vi "Update Hiden Scan Details.vi"(11 "Queue in":refnum<queue>) -> (3 "Queue Out":refnum<queue>)   [LabVIEW 2020]
uses:
  support/Message Queue/Message Cluster.ctl
  support/PCT FGV CMD.ctl
  <instrlib>/Hiden/Public/Scan/Scan Details.ctl
  <instrlib>/Hiden/Public/Scan/Scan Input Details.ctl
  <instrlib>/Hiden/Hiden MS.lvlib
  support/Message Queue/Message Queue.lvlib
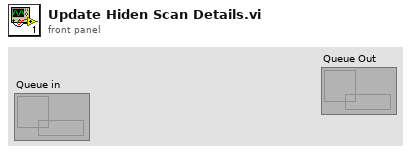
[diagram p1: front panel]
types:
  T1 = cluster{"Input device":string, "Autorange High":i16, "Autorange Low":i16, "Start range":i16, "Dwell (%)":u16, "Settle (%)":u16, "Boolean":bool, "Boolean":bool}
  T2 = typedef "PCT FGV CMD.ctl" = enum16{"INIT", "GET", "SET"}
  T3 = cluster{"Type CMD":string, "Mode CMD":string, "Main CMD":string}
  T4 = typedef "Hiden MS.lvlib/Scan Details.ctl" = cluster{"Device to scan":string, "Start value":dbl, "Stop value":dbl, "Increment":dbl}
  T5 = typedef "Hiden MS.lvlib/Scan Input Details.ctl" = cluster{"Input device":string, "Autorange High":i16, "Autorange Low":i16, "Start range":i16, "Dwell (%)":u16, "Settle (%)":u16, "Dwell is ms?":bool, "Settle is ms?":bool}
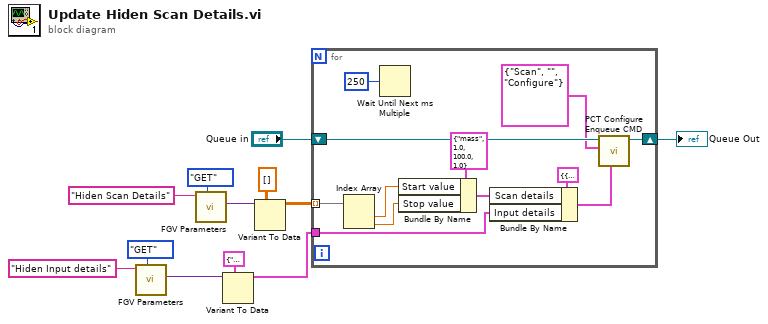
[diagram p0: block diagram]
diagram:
  n1 = call "FGV Parameters.vi"("CMD"=PCT_FGV_CMD."GET", "Key"="Hiden Input details") -> ("output"=w5:variant)  [unwired: 7 in, 2 out]
  n2 = call "FGV Parameters.vi"("CMD"=PCT_FGV_CMD."GET", "Key"="Hiden Scan Details") -> ("output"=w7:variant)  [unwired: 7 in, 2 out]
  n3 = Variant To Data(type=T1 {"Input device"="Faraday", "Autorange High"=-7, "Autorange Low"=-7, "Start range"=-7, "Dwell (%)"=100, "Settle (%)"=100, "Boolean"=FALSE, "Boolean"=FALSE} ("Hiden Input details"), Variant=w5) -> (data=w3:T1)  [unwired: 1 in, 1 out]
  n4 = Variant To Data(type=dbl[][] [] ("Hiden Scan Details"), Variant=w7) -> (data=w6:dbl[][])  [unwired: 1 in, 1 out]
  n5 = for {
    tunnel: w6 -> [w23] mode=indexing
    tunnel: w3 -> [w18]
    shift-right: [w13] -> w1
    shift-left: "Queue in" -> [w17]
    n6 = Index Array(array=w23) -> (element #1=w22:dbl, element #2=w21:dbl)  [unwired: 2 in]
    n7 = Wait Until Next ms Multiple(millisecond multiple=u32 250) -> ()  [unwired: 1 out]
    n8 = Bundle By Name(cluster=T4 {"Device to scan"="mass", "Start value"=1.0, "Stop value"=100.0, "Increment"=1.0} ("Scan details"), "Start value"=w22, "Stop value"=w21) -> (w19:T4)
    n9 = Bundle By Name(cluster=cluster{"Scan details":T4, "Input details":T5} {"Scan details"={"Device to scan"="mass", "Start value"=1.0, "Stop value"=100.0, "Increment"=1.0}, "Input details"={"Input device"="Faraday", "Autorange High"=-5, "Autorange Low"=-10, "Start range"=-7, "Dwell (%)"=100, "Settle (%)"=100, "Dwell is ms?"=FALSE, "Settle is ms?"=FALSE}} ("Scan Config"), "Scan details"=w19, "Input details"=w18) -> (w16:cluster{"Scan details":T4, "Input details":T5})
    n10 = call "PCT Configure Enqueue CMD.vi"("Parameter Data"=w16, "CMD"=T3 {"Type CMD"="Scan", "Mode CMD"="", "Main CMD"="Configure"}, "CMD Queue in"=w17) -> ("CMD Queue out"=w13:refnum<queue>)  [unwired: 6 in, 2 out]
  }
  "Queue Out" <- w1
